vi "Overlay Pattern Matching Results.vi"(6 "Color":u32(colorbox)=16711680, 7 "Group":string, 8 "error in":errorcluster, 10 "Matches":T2(array[cluster]), 11 "Image":T1) -> (0 "error out":errorcluster, 3 "Image Out":T1)   [LabVIEW 2021]
uses:
  <vilib>/vision/Image Controls.llb/IMAQ Image.ctl
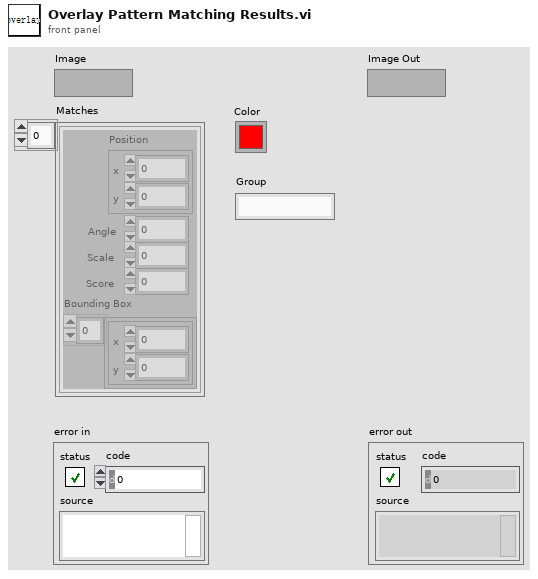
[diagram p1: front panel]
types:
  T1 = typedef "IMAQ Image.ctl" = refnum<image>
  T2 = cluster{"Position":cluster{"x":sgl, "y":sgl}, "Angle":sgl, "Scale":sgl, "Score":sgl, "Bounding Box":cluster{"x":sgl, "y":sgl}[]}[]
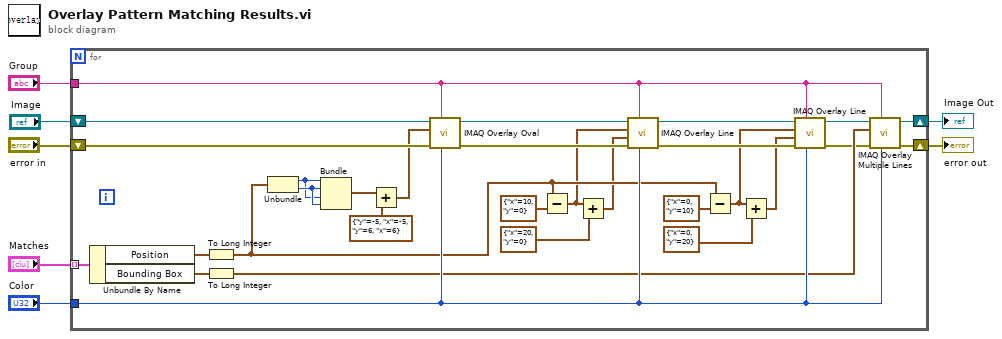
[diagram p0: block diagram]
diagram:
  n1 = for {
    shift-right: [w9] -> w6
    shift-left: "Image" -> [w36]
    tunnel: "Matches" -> [w37] mode=indexing
    tunnel: "Color" -> [w30]
    shift-right: [w33] -> w2
    shift-left: "error in" -> [w34]
    tunnel: "Group" -> [w35]
    n2 = Unbundle By Name(w37) -> ("Position"=w32:cluster{"x":sgl, "y":sgl}, "Bounding Box"=w31:cluster{"x":sgl, "y":sgl}[])
    n3 = To Long Integer(number=w32) -> (32bit integer=w28:cluster{"x":i32, "y":i32})
    n4 = To Long Integer(number=w31) -> (32bit integer=w29:cluster{"x":i32, "y":i32}[])
    n5 = Unbundle(w28) -> ("x"=w12:i32, "y"=w13:i32)
    n6 = Bundle("x"=w12, "y"=w13, "x"=w12, "y"=w13) -> (w14:cluster{"x":i32, "y":i32, "x":i32, "y":i32})  [unwired: 1 out]
    n7 = Add(x=w14, y=cluster{"y":i32, "x":i32, "y":i32, "x":i32} {"y"=-5, "x"=-5, "y"=6, "x"=6}) -> (x+y=w15:cluster{i32, i32, i32, i32})
    n8 = call "IMAQ Overlay Oval"("Color"=w30, "Group"=w35, "error in (no error)"=w34, "Bounding Rectangle"=w15, "Image"=w36) -> ("error out"=w25:errorcluster, "Image Out"=w10:T1)  [unwired: 1 in, 4 out]
    n9 = Subtract(x=w28, y=cluster{"x":i32, "y":i32} {"x"=10, "y"=0}) -> (x-y=w17:cluster{"x":i32, "y":i32})
    n10 = Add(x=w17, y=cluster{"x":i32, "y":i32} {"x"=20, "y"=0}) -> (x+y=w19:cluster{"x":i32, "y":i32})
    n11 = call "IMAQ Overlay Line"("Color"=w30, "Group"=w35, "error in (no error)"=w25, "End Point"=w19, "Start Point"=w17, "Image"=w10) -> ("error out"=w26:errorcluster, "Image Out"=w24:T1)  [unwired: 4 out]
    n12 = Subtract(x=w28, y=cluster{"x":i32, "y":i32} {"x"=0, "y"=10}) -> (x-y=w21:cluster{"x":i32, "y":i32})
    n13 = Add(x=w21, y=cluster{"x":i32, "y":i32} {"x"=0, "y"=20}) -> (x+y=w20:cluster{"x":i32, "y":i32})
    n14 = call "IMAQ Overlay Line"("Color"=w30, "Group"=w35, "error in (no error)"=w26, "End Point"=w20, "Start Point"=w21, "Image"=w24) -> ("error out"=w27:errorcluster, "Image Out"=w11:T1)  [unwired: 4 out]
    n15 = call "IMAQ Overlay Multiple Lines"("Color"=w30, "Group"=w35, "error in (no error)"=w27, "Line End Points"=w29, "Image"=w11) -> ("error out"=w33:errorcluster, "Image Out"=w9:T1)  [unwired: 1 in, 4 out]
  }
  "Image Out" <- w6
  "error out" <- w2
